vi "FIFOStorage.vi"(1 "Set/Get":bool, 2 "Storage Info (input)":cluster{"Store Data":bool, "Destination:":path}) -> (0 "Storage Info (output)":cluster{"Store Data":bool, "Destination:":path})   [LabVIEW 2009]
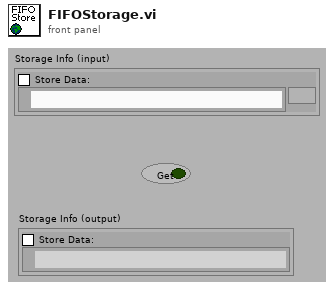
[diagram p1: front panel]
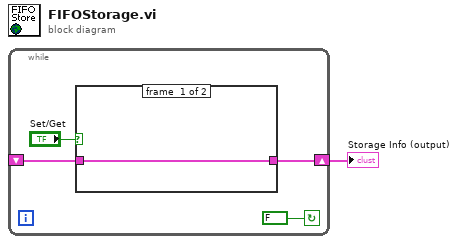
[diagram p0: block diagram]
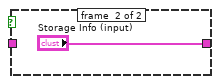
[diagram p2: hidden frame]
diagram:
  n1 = while {
    shift-right: [w3] -> w1
    shift-left: _ -> [w2]
    stop <- FALSE continue-if-true
    n2 = case shown="False" "Set/Get" {
      tunnel: [w6 "Storage Info (input)"] -> w3
      tunnel: w2 -> [w6 _]
      frame #0 {
      }
      frame #1 {
      }
    }
  }
  "Storage Info (output)" <- w1
